vi "Start Write Action.vi"(5 "File Size":u64, 7 "Disk":string, 8 "error in (no error)":errorcluster, 9 "Block Size":u64, 10 "Thread":i32, 11 "File Worker in":refnum<class "File Worker.lvclass">) -> (0 "error out":errorcluster, 3 "File Worker out":refnum<class "File Worker.lvclass">)   [LabVIEW 2025, in "File Worker.lvlib" / "File Worker.lvclass"]
uses:
  File Worker.lvclass
  C:/Program Files/National Instruments/LabVIEW 2025/vi.lib/ActorFramework/Actor/Actor.lvclass
  <vilib>/ActorFramework/Actor/Actor.lvclass/Actor.ctl
  File Worker.lvclass/File Worker.ctl
  Main/Main Messages/Handle Write Speed Msg/Handle Write Speed Msg.lvclass/Handle Write Speed Msg.ctl
  <vilib>/ActorFramework/Message Enqueuer/Message Enqueuer.lvclass/Message Enqueuer.ctl
  Main/Main Messages/Write Done Msg/Write Done Msg.lvclass/Write Done Msg.ctl
  <vilib>/ActorFramework/Message Enqueuer/Enqueue.vi
  Main/Main Messages/Handle Write Speed Msg/Handle Write Speed Msg.lvclass
  C:/Program Files/National Instruments/LabVIEW 2025/vi.lib/ActorFramework/Message/Message.lvclass
  Main/Main Messages/Write Done Msg/Write Done Msg.lvclass
  <vilib>/Utility/tdmsutil.llb/TDMS Generate Random Data (I16).vi
  <vilib>/ActorFramework/Message Priority Queue/Priority Enqueue.vi
  <vilib>/ActorFramework/Actor/Actor.lvclass
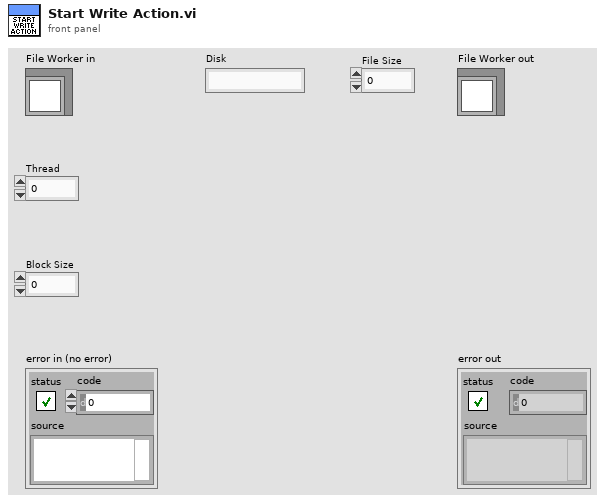
[diagram p1: front panel]
types:
  T1 = enum16{"open", "open or create", "create or replace", "create", "open (read-only)"}
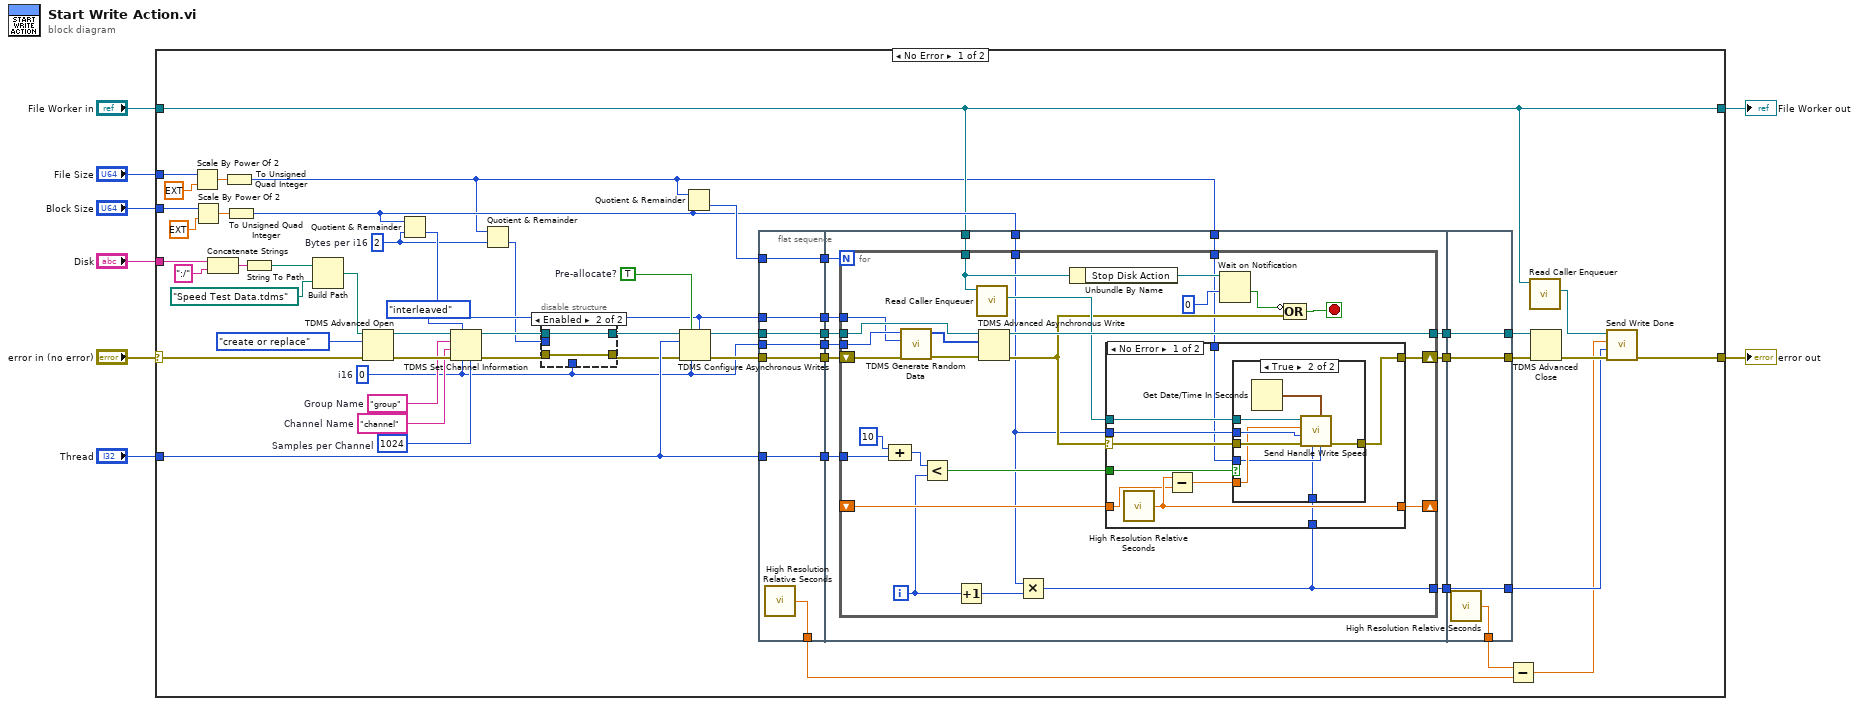
[diagram p0: block diagram]
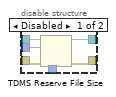
[diagram p2: hidden frame]
diagram:
  n1 = case shown="No Error" "error in (no error)" {
    selector: "error in (no error)" -> [w35 w142]
    tunnel: [w20 w142] -> w7
    tunnel: [w23 w141] -> w5
    tunnel: "File Worker in" -> [w23 w141]
    tunnel: "Disk" -> [w47 _]
    tunnel: "Block Size" -> [w40 _]
    tunnel: "File Size" -> [w43 _]
    tunnel: "Thread" -> [w38 _]
    frame No Error {
      w52 = TRUE  # Pre-allocate?
      w54 = "group"  # Group Name
      w11 = u64 2  # Bytes per i16
      w55 = "channel"  # Channel Name
      w13 = i16 0  # i16
      w58 = u32 1024  # Samples per Channel
      n2 = Scale By Power Of 2(n=w43, x=ext 1.0) -> (x*2^n=w42:ext)
      n3 = Scale By Power Of 2(n=w40, x=ext 1.0) -> (x*2^n=w37:ext)
      n4 = Concatenate Strings(w47, ":/" ("string")) -> (w45:string)
      n5 = To Unsigned Quad Integer(1:w42) -> (0:w12:u64)
      n6 = To Unsigned Quad Integer(1:w37) -> (0:w36:u64)
      n7 = String To Path(string=w45) -> (path=w46:path)
      n8 = Build Path(base path=w46, name or relative path=path "Speed Test Data.tdms") -> (appended path=w48:path)
      n9 = TDMS Advanced Open(8:w35, 10:T1."create or replace" ("operation (0:open)"), 11:w48) -> (0:w57:errorcluster, 3:w56:refnum<k34>)  [unwired: 2 in, 1 out]
      n10 = Quotient & Remainder(x=w36, y=w11) -> (floor(x/y)=w51:u64)  [unwired: 1 out]
      n11 = TDMS Set Channel Information(4:w58, 6:w13, 7:enum16{"non-interleaved", "interleaved"}."interleaved" ("data layout (0:non-interleaved)"), 8:w57, 9:w55, 10:w54, 11:w56) -> (0:w16:errorcluster, 3:w17:refnum<k34>)
      n12 = Quotient & Remainder(x=w12, y=w11) -> (floor(x/y)=w10:u64)  [unwired: 1 out]
      n13 = disable-structure shown="Enabled" {
        disable-tunnel: w17 -> [w68 w70]
        disable-tunnel: w16 -> [w67 w69]
        disable-tunnel: [w66 w70] -> w15
        disable-tunnel: [w65 w69] -> w14
        disable-tunnel: w13 -> [w64 _]
        disable-tunnel: w10 -> [w63 _]
        frame Disabled {
          n14 = TDMS Reserve File Size(6:w64, 8:w67, 10:w63, 11:w68) -> (0:w65:errorcluster, 3:w66:refnum<k34>)  [unwired: 1 in]
        }
        frame Enabled {
        }
      }
      n15 = TDMS Configure Asynchronous Writes(5:w51, 6:w13, 7:w52, 8:w14, 10:w38, 11:w15) -> (0:w53:errorcluster, 3:w62:refnum<k34>)  [unwired: 1 in]
      n16 = Quotient & Remainder(x=w12, y=w36) -> (floor(x/y)=w61:u64)  [unwired: 1 out]
      n17 = flat-sequence {
        tunnel: w38 -> [w72]
        tunnel: w51 -> [w73]
        tunnel: w13 -> [w74]
        tunnel: w53 -> [w75]
        tunnel: w61 -> [w76]
        tunnel: w62 -> [w77]
        tunnel: [w77] -> w34
        tunnel: [w76] -> w33
        tunnel: [w75] -> w32
        tunnel: [w74] -> w31
        tunnel: [w73] -> w30
        tunnel: [w72] -> w29
        tunnel: [w71] -> w24
        tunnel: w23 -> [w82]
        tunnel: w36 -> [w80]
        tunnel: w34 -> [w89]
        tunnel: w33 -> [w88]
        tunnel: w32 -> [w85]
        tunnel: w31 -> [w84]
        tunnel: w30 -> [w83]
        tunnel: w29 -> [w81]
        tunnel: [w87] -> w28
        tunnel: [w86] -> w27
        tunnel: [w79] -> w26
        tunnel: w12 -> [w78]
        tunnel: [w139] -> w59
        tunnel: [w140] -> w60
        tunnel: w28 -> [w140]
        tunnel: w27 -> [w139]
        tunnel: [w138] -> w19
        tunnel: w26 -> [w138]
        tunnel: [w137] -> w25
        frame #0 {
          n18 = call <vilib>:"High Resolution Relative Seconds.vi"() -> ("relative seconds"=w71:dbl)
        }
        frame #1 {
          n19 = for {
            N: w88 -> [_]
            tunnel: [w115] -> w86
            shift-right: [w108] -> w87
            shift-left: w85 -> [w113]
            tunnel: w89 -> [w112]
            tunnel: w84 -> [w110]
            tunnel: w83 -> [w104]
            tunnel: w82 -> [w101]
            tunnel: w81 -> [w96]
            shift-right: [w106] -> _
            shift-left: _ -> [w105]
            tunnel: w80 -> [w93]
            tunnel: [w91] -> w79
            tunnel: w78 -> [w94]
            i -> [w92]
            stop <- w102 stop-if-true
            n20 = Compound Arithmetic op=unknown(10 ("value"), w96) -> (w97:i32)
            n21 = call-poly <vilib>:"TDMS Generate Random Data.vi"("error in (no error)"=w113, "number of samples"=w104, "data type"=w110) -> ("error out"=w114:errorcluster, "data"=w111:i16[])  [unwired: 7 in]
            n22 = Less?(x=w97, y=w92) -> (x < y?=w107:bool)
            n23 = Increment(x=w92) -> (x+1=w90:i32)
            n24 = call <vilib>:"Read Caller Enqueuer.vi"("Actor"=w101) -> ("Caller Enqueuer"=w109:refnum<class "Message Enqueuer.lvclass">)  [unwired: 10 in]
            n25 = TDMS Advanced Asynchronous Write(8:w114, 10:w111, 11:w112) -> (0:w103:errorcluster, 3:w115:refnum<k34>)
            n26 = Multiply(x=w93, y=w90) -> (x*y=w91:u64)
            n27 = Unbundle By Name(w101) -> ("Stop Disk Action"=w100:refnum<notifier>)
            n28 = case shown="No Error" w103 {
              selector: w103 -> [w124 w136]
              tunnel: w109 -> [w125 _]
              tunnel: [w123 w136] -> w108
              tunnel: w107 -> [w122 _]
              tunnel: [w121 w135] -> w106
              tunnel: w105 -> [w120 w135]
              tunnel: w93 -> [w119 _]
              tunnel: w94 -> [w117 _]
              tunnel: w91 -> [w116 _]
              frame No Error {
                n29 = call <vilib>:"High Resolution Relative Seconds.vi"() -> ("relative seconds"=w121:dbl)
                n30 = Subtract(x=w121, y=w120) -> (x-y=w118:dbl)
                n31 = case shown="True" w122 {
                  tunnel: w125 -> [_ w134]
                  tunnel: w124 -> [w126 w133]
                  tunnel: [w126 w132] -> w123
                  tunnel: w118 -> [_ w129]
                  tunnel: w119 -> [_ w131]
                  tunnel: w117 -> [_ w128]
                  tunnel: w116 -> [_ w127]
                  frame False {
                  }
                  frame True {
                    n32 = Get Date/Time In Seconds() -> (seconds since 1Jan1904=w130:timestamp)
                    n33 = call "Send Handle Write Speed.vi"("Total Bytes"=w128, "Time Stamp"=w130, "Bytes Done"=w127, "error in (no error)"=w133, "Size"=w131, "Time"=w129, "Message Enqueuer"=w134) -> ("error out"=w132:errorcluster)  [unwired: 3 in, 1 out]
                  }
                }
              }
              frame Error {
              }
            }
            n34 = Wait on Notification(notifier=w100, timeout in ms (-1)=0) -> (timed out?=w98:bool)  [unwired: 2 in, 3 out]
            n35 = Compound Arithmetic op=OR(invert w98, w103) -> (w102:bool)
          }
        }
        frame #2 {
          n36 = call <vilib>:"High Resolution Relative Seconds.vi"() -> ("relative seconds"=w137:dbl)
        }
      }
      n37 = Subtract(x=w25, y=w24) -> (x-y=w18:dbl)
      n38 = call <vilib>:"Read Caller Enqueuer.vi"("Actor"=w23) -> ("Caller Enqueuer"=w22:refnum<class "Message Enqueuer.lvclass">)  [unwired: 10 in]
      n39 = TDMS Advanced Close(8:w60, 11:w59) -> (0:w21:errorcluster)  [unwired: 2 in, 1 out]
      n40 = call "Send Write Done.vi"("error in (no error)"=w21, "Bytes"=w19, "Time"=w18, "Message Enqueuer"=w22) -> ("error out"=w20:errorcluster)  [unwired: 6 in, 1 out]
    }
    frame Error {
    }
  }
  "error out" <- w7
  "File Worker out" <- w5
